vi "ControlValueArrayToJSON.vi"(7 "UseEnum":bool, 8 "error in (no error)":errorcluster, 9 "Array in":variant, 11 "Control in":refnum<vi>) -> (0 "error out":errorcluster, 3 "String out":string)   [LabVIEW 2019]
uses:
  <vilib>/Utility/Data Type/NI_Data Type.lvlib
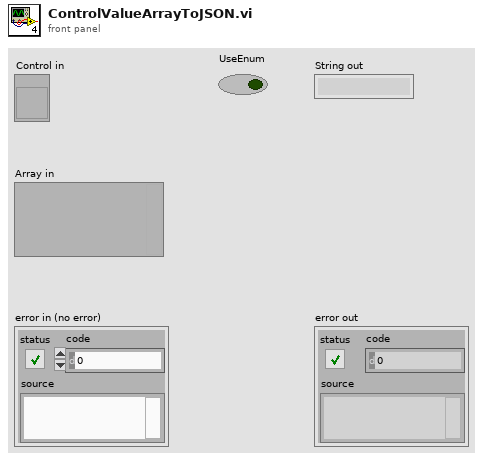
[diagram p1: front panel]
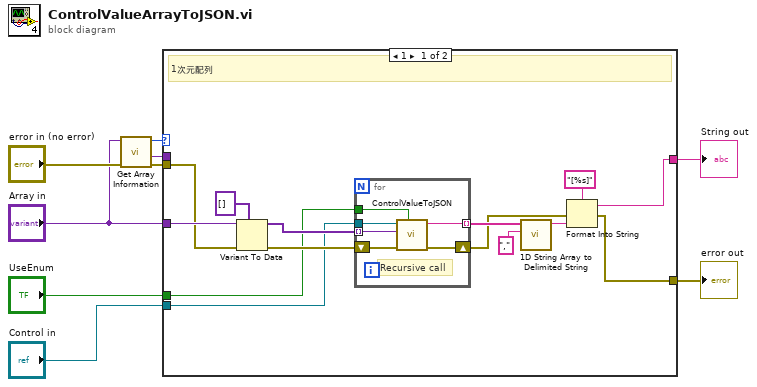
[diagram p0: block diagram]
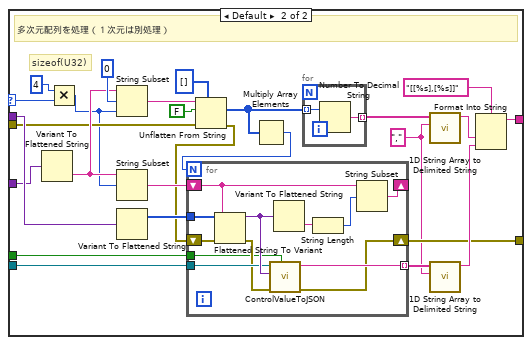
[diagram p2: hidden frame]
diagram:
  n1 = call <vilib>:"Get Array Information.vi"("error in (no error)"="error in (no error)", "variant"="Array in") -> ("error out"=w5:errorcluster, "array element data type"=w9:variant, "number of dimensions"=w2:i32)  [unwired: 6 in, 1 out]
  n2 = case shown="1" w2 {
    selector: w2 -> [_ w35]
    tunnel: w9 -> [_ w46]
    tunnel: "Control in" -> [w14 w44]
    tunnel: [w13 w40] -> w7
    tunnel: w5 -> [w11 w39]
    tunnel: [w12 w37] -> w4
    tunnel: "Array in" -> [w15 w36]
    tunnel: "UseEnum" -> [w10 w34]
    frame 1 {
      # "1次元配列"
      n3 = Variant To Data(error in=w11, type=variant[] [], Variant=w15) -> (data=w23:variant[], error out=w18:errorcluster)
      n4 = for {
        tunnel: w23 -> [w29] mode=indexing
        tunnel: [w28] -> w22 mode=indexing
        shift-right: [w26] -> w17
        shift-left: w18 -> [w27]
        tunnel: w14 -> [w25]
        tunnel: w10 -> [w24]
        # "Recursive call"
        n5 = call "ControlValueToJSON.vi"("UseEnum"=w24, "error in (no error)"=w27, "Value"=w29, "Control in"=w25) -> ("error out"=w26:errorcluster, "String"=w28:string)  [unwired: 6 in]
      }
      n6 = call <vilib>:"1D String Array to Delimited String.vi"("delimiter"=",", "string array"=w22) -> ("delimited string"=w20:string)  [unwired: 9 in]
      n7 = Format Into String(format string="[%s]", error in=w17, w20) -> (resulting string=w13:string, error out=w12:errorcluster)  [unwired: 1 in]
    }
    frame Default {
      w30 = "," ("delimiter")
      # "sizeof(U32)"
      # "多次元配列を処理（１次元は別処理）"
      n8 = Variant To Flattened String(Variant=w36) -> (data string=w53:string)  [unwired: 1 out]
      n9 = Multiply(x=4, y=w35) -> (x*y=w33:i32)
      n10 = String Subset(string=w53, offset (0)=0, length (rest)=w33) -> (substring=w52:string)
      n11 = String Subset(string=w53, offset (0)=w33) -> (substring=w47:string)  [unwired: 1 in]
      n12 = Variant To Flattened String(Variant=w46) -> (1:w45:i16[])  [unwired: 1 out]
      n13 = Unflatten From String(type=i32[] [], binary string=w52, data includes array or string size? (T)=FALSE, error in (no error)=w39) -> (value=w32:i32[], error out=w38:errorcluster)  [unwired: 1 in, 1 out]
      n14 = Multiply Array Elements(1:w32) -> (0:w31:i32)
      n15 = for {
        N: w31 -> [_]
        shift-right: [w65] -> _
        shift-left: w47 -> [w64]
        tunnel: w45 -> [w67]
        tunnel: w44 -> [w61]
        tunnel: [w60] -> w43 mode=indexing
        shift-right: [w57] -> w37
        shift-left: w38 -> [w59]
        tunnel: w34 -> [w56]
        n16 = Flattened String To Variant(4:w59, 6:w64, 7:w67) -> (0:w58:errorcluster, 3:w62:variant)
        n17 = call "ControlValueToJSON.vi"("UseEnum"=w56, "error in (no error)"=w58, "Value"=w62, "Control in"=w61) -> ("error out"=w57:errorcluster, "String"=w60:string)  [unwired: 6 in]
        n18 = Variant To Flattened String(Variant=w62) -> (data string=w66:string)  [unwired: 1 out]
        n19 = String Length(string=w66) -> (length=w63:i32)
        n20 = String Subset(string=w64, offset (0)=w63) -> (substring=w65:string)  [unwired: 1 in]
      }
      n21 = for {
        tunnel: w32 -> [w68] mode=indexing
        tunnel: [w69] -> w49 mode=indexing
        n22 = Number To Decimal String(number=w68) -> (decimal integer string=w69:string)  [unwired: 1 in]
      }
      n23 = call <vilib>:"1D String Array to Delimited String.vi"("delimiter"=w30, "string array"=w49) -> ("delimited string"=w41:string)  [unwired: 9 in]
      n24 = call <vilib>:"1D String Array to Delimited String.vi"("delimiter"=w30, "string array"=w43) -> ("delimited string"=w42:string)  [unwired: 9 in]
      n25 = Format Into String(format string="[[%s],[%s]]", w41, w42) -> (resulting string=w40:string)  [unwired: 2 in, 1 out]
    }
  }
  "error out" <- w4
  "String out" <- w7
